vi "Read RC parameters_override_UI.vi"(0 "JSON FilePath":path=path "F:/User Interface Testbench/Configuration file/Rack Controller Override JSON UI.json", 1 "ListBox Cluster":T1, 5 "Rack Id":string="0", 7 "Variant":variant, 9 "Part Name":string, 11 "error in (no error)":errorcluster, 12 "Variant?":bool) -> (4 "Output Edit Tolerance cluster":T1, 6 "Error Message":string, 15 "error out":errorcluster)   [LabVIEW 2019, in "ZenGage v3.0 UI.lvclass"]
uses:
  ZenGage v3.0 UI.lvclass
  Type Definitions/JSON Read/Rack controller json override.ctl
  Type Definitions/Edit tolerance settings/Rack Selection.ctl
  <vilib>/Utility/miscctls.llb/LVPoint32TypeDef.ctl
  Type Definitions/Edit tolerance settings/Edit Tolerance Input.ctl
panel:
  out "VCluster\n out":variant
  # "e"
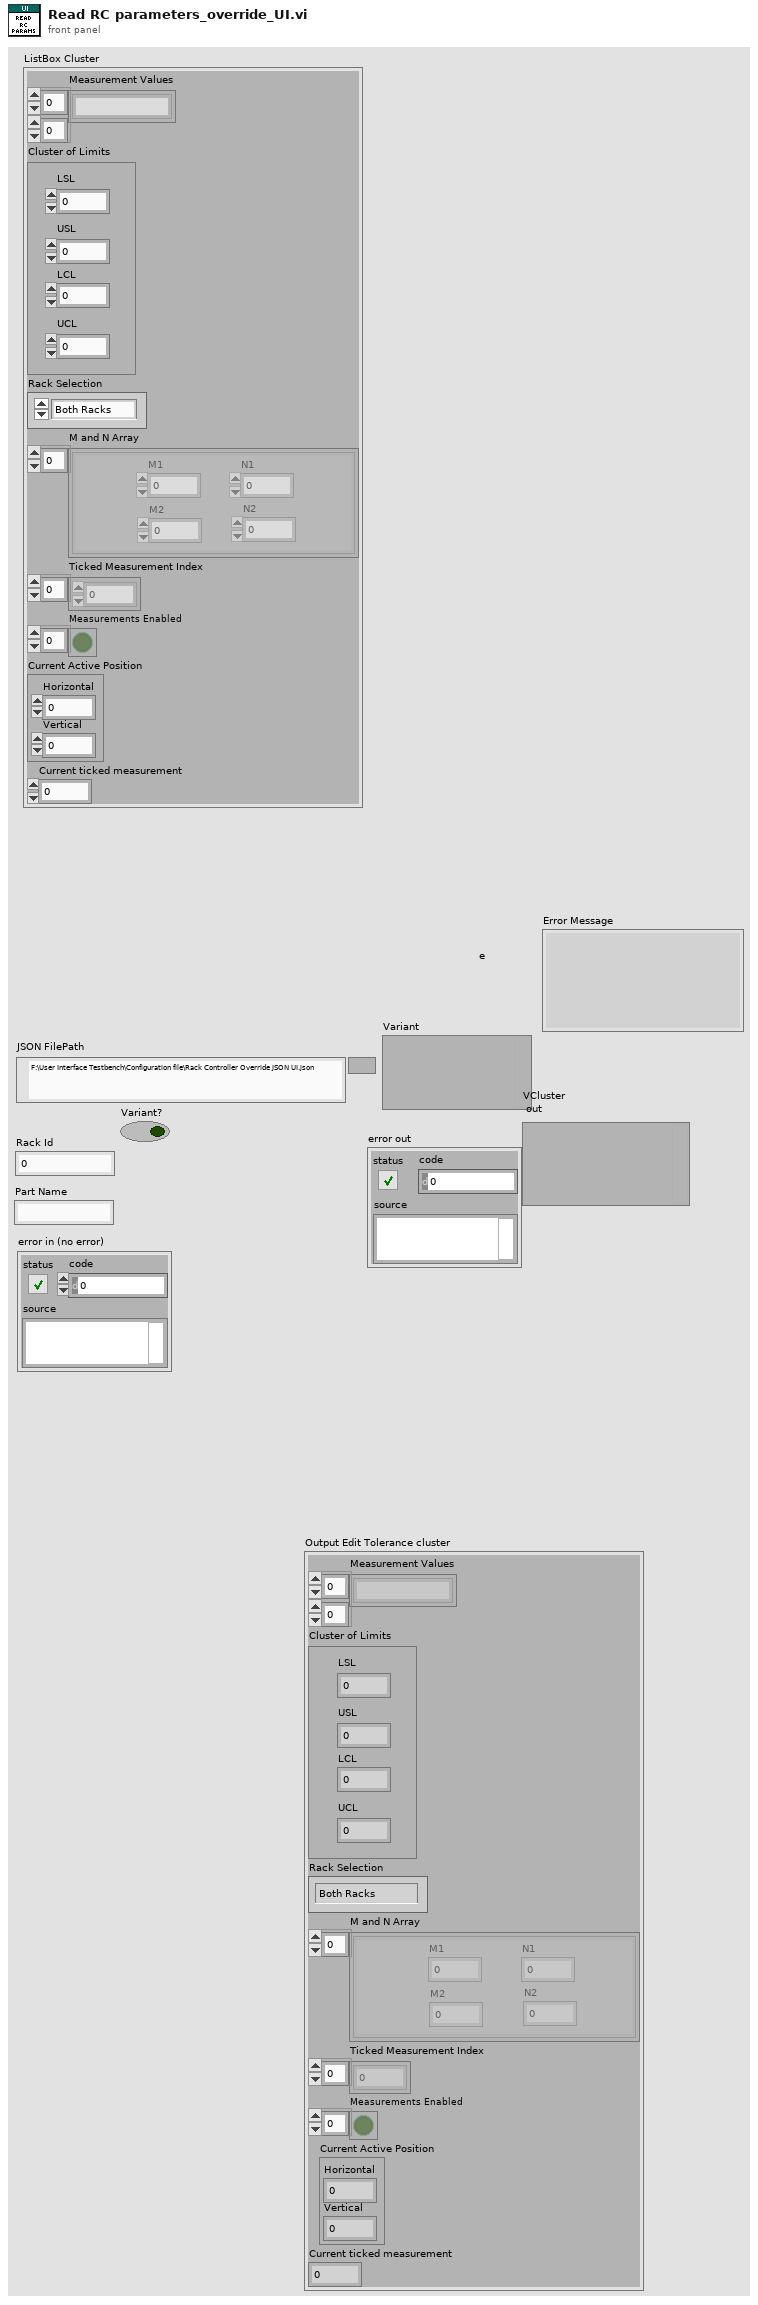
[diagram p1: front panel]
types:
  T1 = typedef "ZenGage v3.0 UI.lvclass/Edit Tolerance Input.ctl" = cluster{"Measurement Values":string[][], "Cluster of Limits":cluster{"LSL":dbl, "USL":dbl, "LCL":dbl, "UCL":dbl}, "Rack Selection":T2, "M and N Array":cluster{"M1":u64, "M2":u64, "N1":u64, "N2":u64}[], "Ticked Measurement Index":u32[], "Measurements Enabled":bool[], "Current Active Position":T3, "Current ticked measurement":dbl}
  T2 = typedef "ZenGage v3.0 UI.lvclass/Rack Selection.ctl" = enum16{"Both Racks", "Rack 2", "Rack 1"}
  T3 = typedef "LVPoint32TypeDef.ctl" = cluster{"Horizontal":i32, "Vertical":i32}
  T4 = typedef "Rack controller json override.ctl" = cluster{"RackControllerParameters":cluster{"RackId":dbl, "PartsList":cluster{"Name":string, "Measurements":cluster{"MeasurementId":dbl, "Name":string, "MeasurementEnable":bool, "ControlLimitsViolationThreshold":cluster{"AllowableFails":dbl, "WindowSize":dbl}, "SpecificationLimitViolationThreshold":cluster{"AllowableFails":dbl, "WindowSize":dbl}}[]}[]}[]}
  T5 = cluster{"RackId":dbl, "PartsList":cluster{"Name":string, "Measurements":cluster{"MeasurementId":dbl, "Name":string, "MeasurementEnable":bool, "ControlLimitsViolationThreshold":cluster{"AllowableFails":dbl, "WindowSize":dbl}, "SpecificationLimitViolationThreshold":cluster{"AllowableFails":dbl, "WindowSize":dbl}}[]}[]}[]
  T6 = cluster{"RackId":dbl, "PartsList":cluster{"Name":string, "Measurements":cluster{"MeasurementId":dbl, "Name":string, "MeasurementEnable":bool, "ControlLimitsViolationThreshold":cluster{"AllowableFails":dbl, "WindowSize":dbl}, "SpecificationLimitViolationThreshold":cluster{"AllowableFails":dbl, "WindowSize":dbl}}[]}[]}
  T7 = cluster{"Name":string, "Measurements":cluster{"MeasurementId":dbl, "Name":string, "MeasurementEnable":bool, "ControlLimitsViolationThreshold":cluster{"AllowableFails":dbl, "WindowSize":dbl}, "SpecificationLimitViolationThreshold":cluster{"AllowableFails":dbl, "WindowSize":dbl}}[]}[]
  T8 = cluster{"Name":string, "Measurements":cluster{"MeasurementId":dbl, "Name":string, "MeasurementEnable":bool, "ControlLimitsViolationThreshold":cluster{"AllowableFails":dbl, "WindowSize":dbl}, "SpecificationLimitViolationThreshold":cluster{"AllowableFails":dbl, "WindowSize":dbl}}[]}
  T9 = cluster{cluster{"Name":string, "Measurements":cluster{"MeasurementId":dbl, "Name":string, "MeasurementEnable":bool, "ControlLimitsViolationThreshold":cluster{"AllowableFails":dbl, "WindowSize":dbl}, "SpecificationLimitViolationThreshold":cluster{"AllowableFails":dbl, "WindowSize":dbl}}[]}}
  T10 = cluster{"MeasurementId":dbl, "Name":string, "MeasurementEnable":bool, "ControlLimitsViolationThreshold":cluster{"AllowableFails":dbl, "WindowSize":dbl}, "SpecificationLimitViolationThreshold":cluster{"AllowableFails":dbl, "WindowSize":dbl}}[]
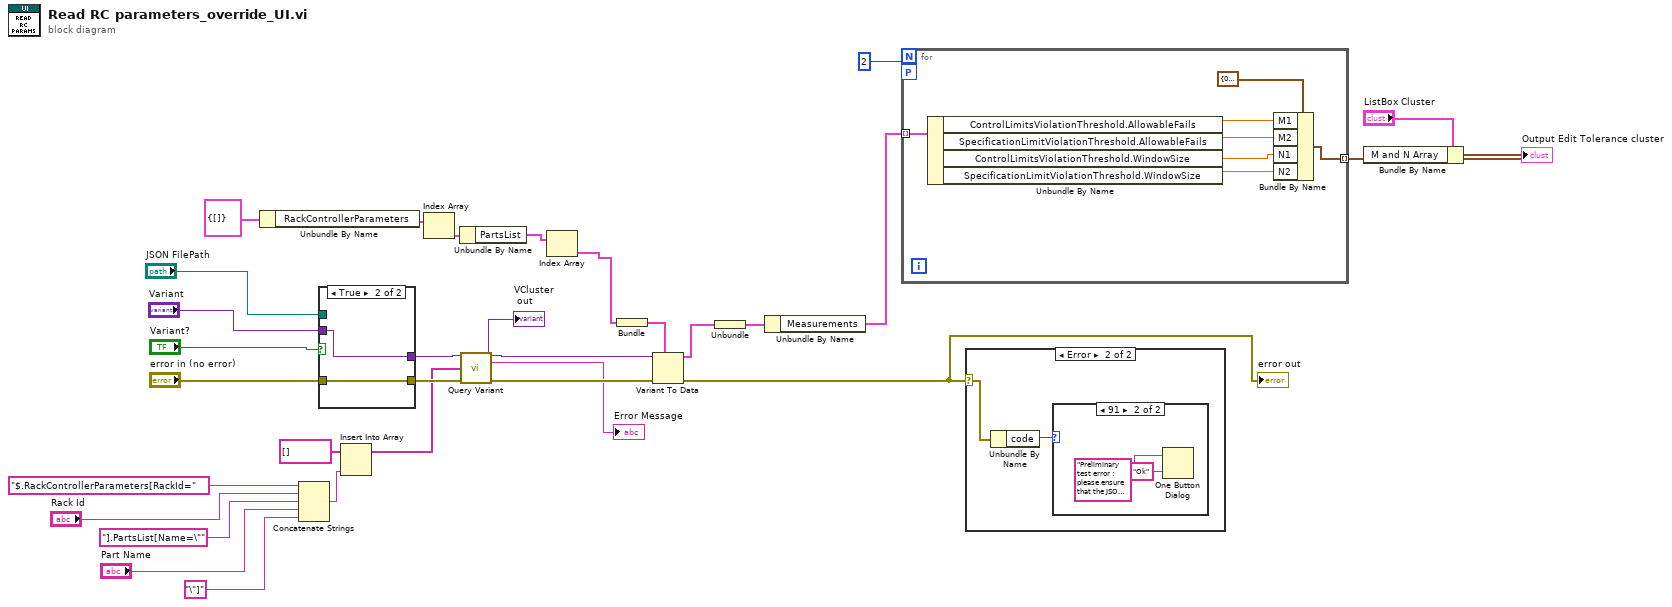
[diagram p0: block diagram]
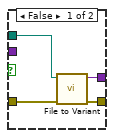
[diagram p4: hidden frame]
diagram:
  n1 = Unbundle By Name(T4 {"RackControllerParameters"=[]}) -> ("RackControllerParameters"=w4:T5)
  n2 = Concatenate Strings("$.RackControllerParameters[RackId=" ("string"), "Rack Id", "].PartsList[Name=\"" ("string"), "Part Name", "\"]" ("string")) -> (w19:string)
  n3 = case shown="True" "Variant?" {
    tunnel: [w35 w37] -> w31
    tunnel: "error in (no error)" -> [w34 w37]
    tunnel: [w33 w36] -> w27
    tunnel: "JSON FilePath" -> [w32 _]
    tunnel: "Variant" -> [_ w36]
    frame False {
      n4 = call <vilib>:"File to Variant.vi"("JSON FilePath"=w32, "error in (no error)"=w34) -> ("JSON Variant"=w33:variant, "error out"=w35:errorcluster)  [unwired: 6 in, 1 out]
    }
    frame True {
    }
  }
  n5 = Insert Into Array(array=string[] [], new element=w19) -> (w17:string[])  [unwired: 1 in]
  n6 = Index Array(array=w4) -> (element=w3:T6)  [unwired: 1 in]
  n7 = Unbundle By Name(w3) -> ("PartsList"=w2:T7)
  n8 = call <vilib>:"Query Variant.vi"("VCluster in"=w27, "pathList"=w17, "error IO"=w31) -> ("VCluster\n out"=w28:variant, "Error Message"=→"Error Message":string, "error out"=w29:errorcluster)  [unwired: 9 in, 1 out]
  "VCluster\n out" <- w28
  n9 = Index Array(array=w2) -> (element=w1:T8)  [unwired: 1 in]
  n10 = Bundle(w1) -> (w9:T9)  [unwired: 1 in]
  n11 = Variant To Data(error in=w29, type=w9, Variant=w28) -> (data=w8:T9, error out=w6:errorcluster)
  "error out" <- w6
  n12 = Unbundle(w8) -> (w10:T8)
  n13 = Unbundle By Name(w10) -> ("Measurements"=w15:T10)
  n14 = for {
    tunnel: w15 -> [w44] mode=indexing
    tunnel: [w38] -> w14 mode=indexing
    workers-P: 2 -> [_]
    n15 = Unbundle By Name(w44) -> ("ControlLimitsViolationThreshold.AllowableFails"=w42:dbl, "SpecificationLimitViolationThreshold.AllowableFails"=w41:dbl, "ControlLimitsViolationThreshold.WindowSize"=w40:dbl, "SpecificationLimitViolationThreshold.WindowSize"=w39:dbl)
    n16 = Bundle By Name(cluster=cluster{"M1":u64, "M2":u64, "N1":u64, "N2":u64} {"M1"=0, "M2"=0, "N1"=0, "N2"=0} ("Rack 1"), "M1"=w42, "M2"=w41, "N1"=w40, "N2"=w39) -> (w38:cluster{"M1":u64, "M2":u64, "N1":u64, "N2":u64})
  }
  n17 = case shown="Error" w6 {
    selector: w6 -> [_ w46]
    frame No Error {
    }
    frame Error {
      n18 = Unbundle By Name(w46) -> ("code"=w45:i32)
      n19 = case shown="91" w45 {
        frame 0, Default {
        }
        frame 91 {
          n20 = One Button Dialog(message="Preliminary test error : please ensure that the JSON configuration structure has not been modified. If yes, then please modify the Rack controller override typedef in the user interface module.\nIt is recommended to exit the software now. ", button name ("OK")="Ok") -> ()  [unwired: 1 out]
        }
      }
    }
  }
  n21 = Bundle By Name(cluster="ListBox Cluster", "M and N Array"=w14) -> (→"Output Edit Tolerance cluster":T1)
